vi "Launcher.vi"   [LabVIEW 2019]
uses:
  FirstAF.lvclass
  C:/Program Files (x86)/National Instruments/LabVIEW 2019/vi.lib/ActorFramework/Actor/Actor.lvclass
  <vilib>/ActorFramework/Actor/Actor.lvclass
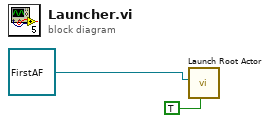
[diagram p0: block diagram]
diagram:
  n1 = call <vilib>:"Launch Root Actor.vi"("Open Actor Core front panel? (F)"=TRUE, "Actor"=refnum<class "FirstAF.lvclass"> refnum ("FirstAF.lvlib:FirstAF.lvclass")) -> ()  [unwired: 8 in, 2 out]
